vi "JDP-JSON Test Marshall-Unmarshall.vi"() -> ()   [LabVIEW 2019]
uses:
  Test Cluster.ctl
  Serializer.JDP-JSON.lvclass
  C:/Program Files (x86)/National Instruments/LabVIEW 2019/vi.lib/LabVIEW Open Source Project/OpenSerializer/Serializer/Serializer.lvclass
  Serializer.JDP-JSON.lvclass/Serializer.JDP-JSON.ctl
  Write Enable LV Extensions.vi
  Write Pretty Print.vi
  <vilib>/LabVIEW Open Source Project/OpenSerializer/Serializer/Serializer.lvclass
panel:
  out "Pass?":bool
  out "Data Cluster out":T1={"Boolean"=FALSE, "String"="", "Path"=path "", "Numeric"=0.0, "Enum"=enum."Item0", "Array"=[], "Sub-Cluster"={"Numeric"=0.0, "Boolean"=FALSE, "String"=""}} {"Numeric" format="%#_10g"}
  out "JSON String":string
  in  "Pretty Print":bool=TRUE
  in  "Enable LV Extensions":bool=TRUE
  in  "Data Cluster in":T1={"Boolean"=TRUE, "String"="Test String Here", "Path"=path "C:/Windows", "Numeric"=3.141592654, "Enum"=enum."Item0", "Array"=[0.0, 1.0, 2.0, 3.0, 4.0, 5.0, 6.0], "Sub-Cluster"={"Numeric"=4.0, "Boolean"=FALSE, "String"="Another test string"}} {"Numeric" format="%#_10g"}
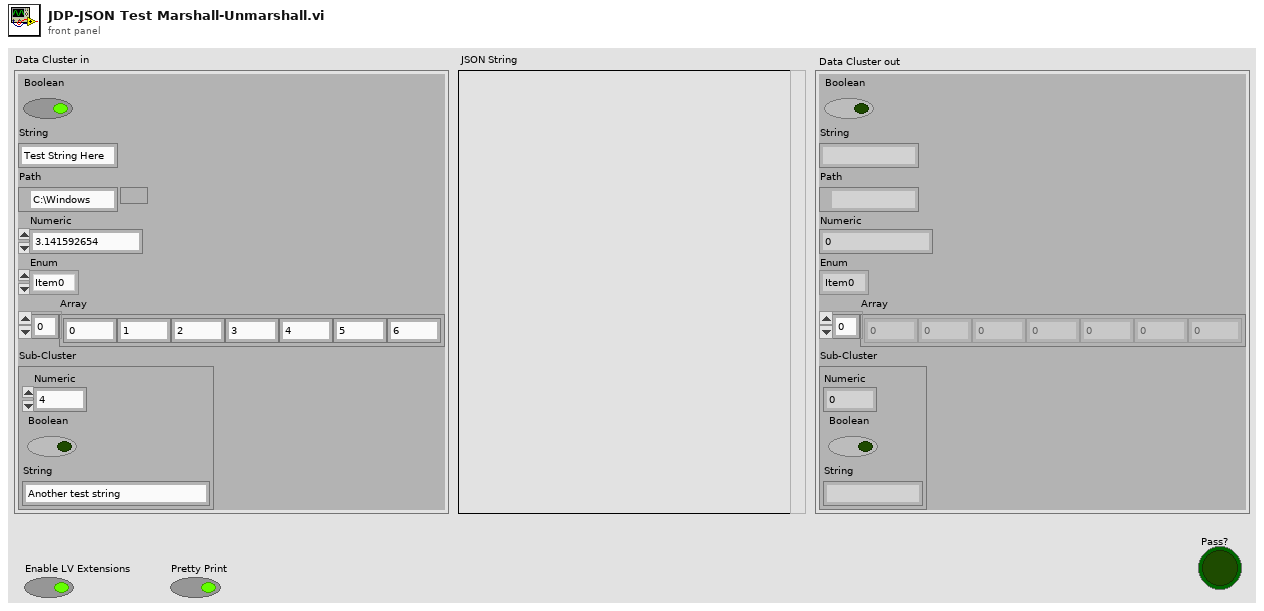
[diagram p1: front panel]
types:
  T1 = typedef "Test Cluster.ctl" = cluster{"Boolean":bool, "String":string, "Path":path, "Numeric":dbl, "Enum":enum16{"Item0", "Item1"}, "Array":dbl[], "Sub-Cluster":cluster{"Numeric":dbl, "Boolean":bool, "String":string}}
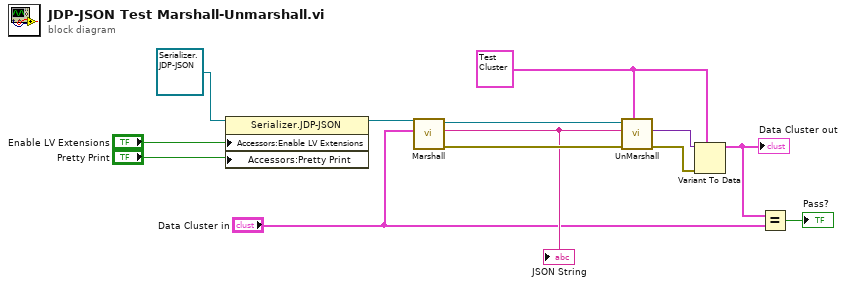
[diagram p0: block diagram]
diagram:
  w4 = T1 {"Boolean"=FALSE, "String"="", "Path"=path "", "Numeric"=0.0, "Enum"=enum."Item0", "Array"=[], "Sub-Cluster"={"Numeric"=0.0, "Boolean"=FALSE, "String"=""}} ("Cluster")
  n1 = property class="Serializer.JDP-JSON"(reference=refnum<class "Serializer.JDP-JSON.lvclass"> refnum ("OpenSerializer.JDP-JSON.lvlib:Serializer.JDP-JSON.lvclass"), "Accessors:Enable LV Extensions"="Enable LV Extensions", "Accessors:Pretty Print"="Pretty Print") -> (reference out=w8:refnum<class "Serializer.JDP-JSON.lvclass">)  [unwired: 1 in, 1 out]
  n2 = call <vilib>:"Marshall.vi"("Variant"="Data Cluster in", "Serializer in"=w8) -> ("error out"=w13:errorcluster, "String"=w7:string, "Serializer out"=w12:refnum<class "Serializer.JDP-JSON.lvclass">)  [unwired: 7 in]
  "JSON String" <- w7
  n3 = call <vilib>:"UnMarshall.vi"("Type"=w4, "error in (no error)"=w13, "String"=w7, "Serializer in"=w12) -> ("error out"=w6:errorcluster, "Variant"=w5:variant)  [unwired: 5 in, 1 out]
  n4 = Variant To Data(error in=w6, type=w4, Variant=w5) -> (data=w3:T1)  [unwired: 1 out]
  "Data Cluster out" <- w3
  n5 = Equal?(x=w3, y="Data Cluster in") -> (x = y?=→"Pass?":bool)
